vi "SubVI_TDMSfile_anal.vi"() -> (3 "file path out":path caption="파일 경로 출력")   [LabVIEW 2016]
uses:
  <vilib>/Utility/tdmsutil.llb/fileViewerConfigData.ctl
  <vilib>/Utility/error.llb/DialogType.ctl
  <vilib>/event_ctls.llb/sizeaction.ctl
  <vilib>/event_ctls.llb/panelstate.ctl
  <vilib>/Utility/tdmsutil.llb/TDMSFileViewerLocalizedText.vi
panel:
  out "Resize?":bool caption="크기 조정?"
  in  "Quit":bool caption="종료"
  in  "File contents":string(tree) caption="파일 내용"
  in  "Settings...":bool caption="셋팅..."
  in  "Status":string caption="상태"
  in  "Help":bool caption="도움말"
  in  "LastTopLeftValue":u64 caption="마지막 왼쪽 위 값"
  out "Temp Configuration":T1 caption="임시 설정"
  out "TotalCount":u64 caption="전체 카운트"
  out "error out":errorcluster caption="에러 출력"
  in  "error in (no error)":errorcluster caption="에러 입력(에러 없음)"
  in  "file path":path caption="파일 경로"
  in  "Properties / Values / Graph":T2(tab) caption="프로퍼티 / 값 / 그래프"
  in  "Properties":i32(listbox) caption="프로퍼티"
  in  "Go To":bool caption="이동하기"
  in  "Scrollbar":u64(c297) caption="스크롤 막대"
  in  "Raw data values":i32(listbox) caption="원시 데이터 값"
  out "dt":dbl
  out "Waveform Graph":waveform(dbl)[](graph) caption="웨이브폼 그래프"
  # "1...1000의 값을 디스플레이하기"
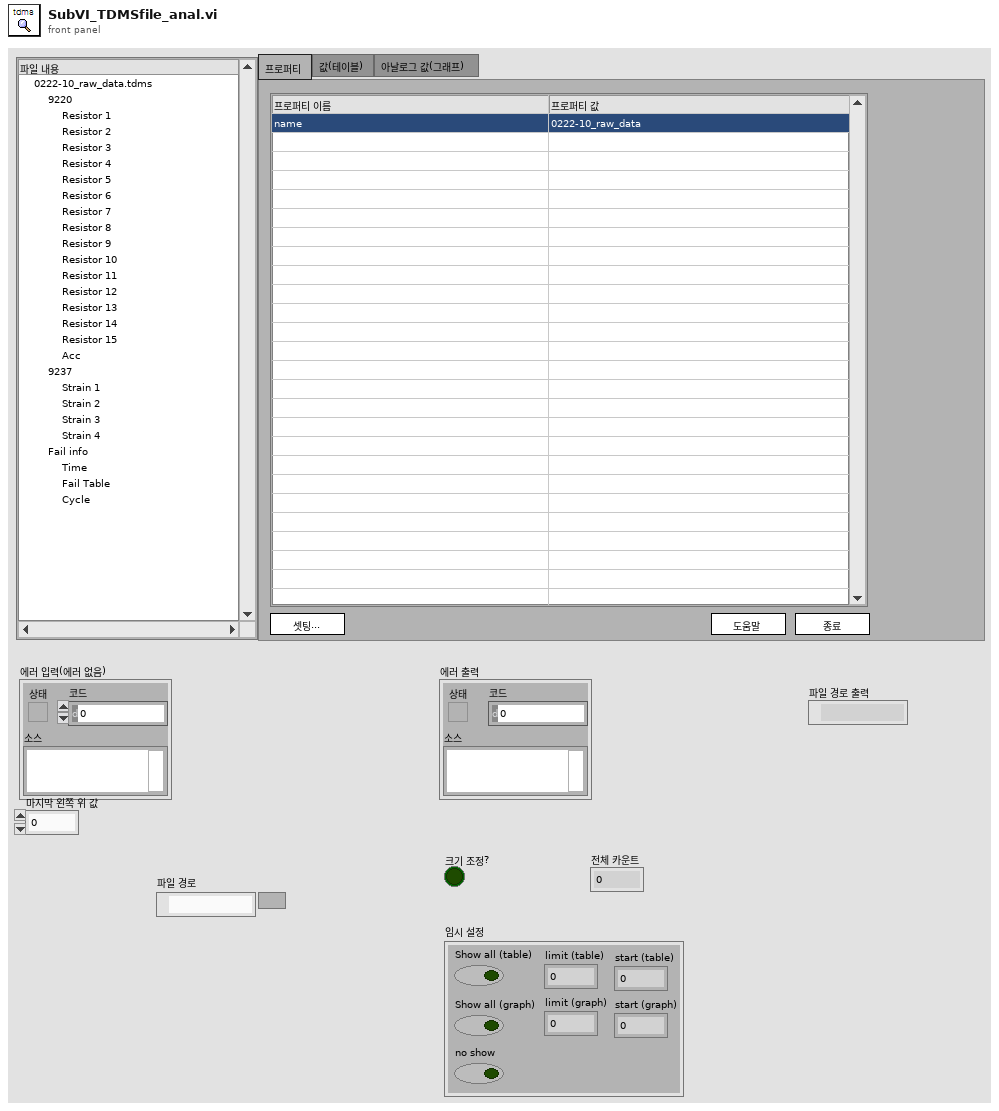
[diagram p1: front panel]
types:
  T1 = typedef "fileViewerConfigData.ctl" = cluster{"Show all (table)":bool, "Show all (graph)":bool, "limit (table)":u64, "limit (graph)":u64, "no show":bool, "start (table)":u64, "start (graph)":u64}
  T2 = enum32{"Properties", "Values (table)", "Analog values (graph)"}
  T3 = enum16{"open", "open or create", "create or replace", "create", "open (read-only)"}
  T4 = cluster{"Tree":refnum<vi>, "Tab Control":refnum<vi>, "property list":refnum<vi>, "raw data list":refnum<vi>, "Waveform Graph":refnum<vi>, "Ok":refnum<vi>, "Ok 2":refnum<vi>, "Ok 3":refnum<vi>, "Ok 4":refnum<vi>, "Scrollbar":refnum<vi>, "Ok 5":refnum<vi>, "TopLeftValue":refnum<vi>, "TotalCount":refnum<vi>}
  T5 = typedef "panelstate.ctl" = enum32{"Standard", "Minimized", "Maximized"}
  T6 = typedef "sizeaction.ctl" = enum32{"Minimized", "Maximized", "Resized"}
  T7 = cluster{"Shift":bool, "Ctrl":bool, "Alt":bool, "Cmd":bool, "Opt":bool}
  T8 = typedef "LVRectTypeDef.ctl" = cluster{"Left":i16, "Top":i16, "Right":i16, "Bottom":i16}
  T9 = typedef "LVRowAndColumnUnsignedTypeDef.ctl" = cluster{"Row":u32, "Column":u32}
  T10 = typedef "DialogType.ctl" = u16
  T11 = typedef "eventvkey.ctl" = enum16{"ASCII", "Enter", "Return", "Shift", "Ctrl", "Alt", "Cmd", "Opt", "Caps", "NumLock", "Clear", "Break", "Up", "Down", "Left", "Right", "Insert", "Delete", "Home", "End", "PageUp", "PageDown", "Escape", "Help", "Pause", "ScrollLock", "F1", "F2", "F3", "F4", "F5", "F6", "F7", "F8", "F9", "F10", "F11", "F12", "F13", "F14", "F15", "F16", "F17", "F18", "F19", "F20", "F21", "F22", "F23", "F24", "Play", "VolumeUp", "VolumeDown", "Mute", "Two Byte Char"}
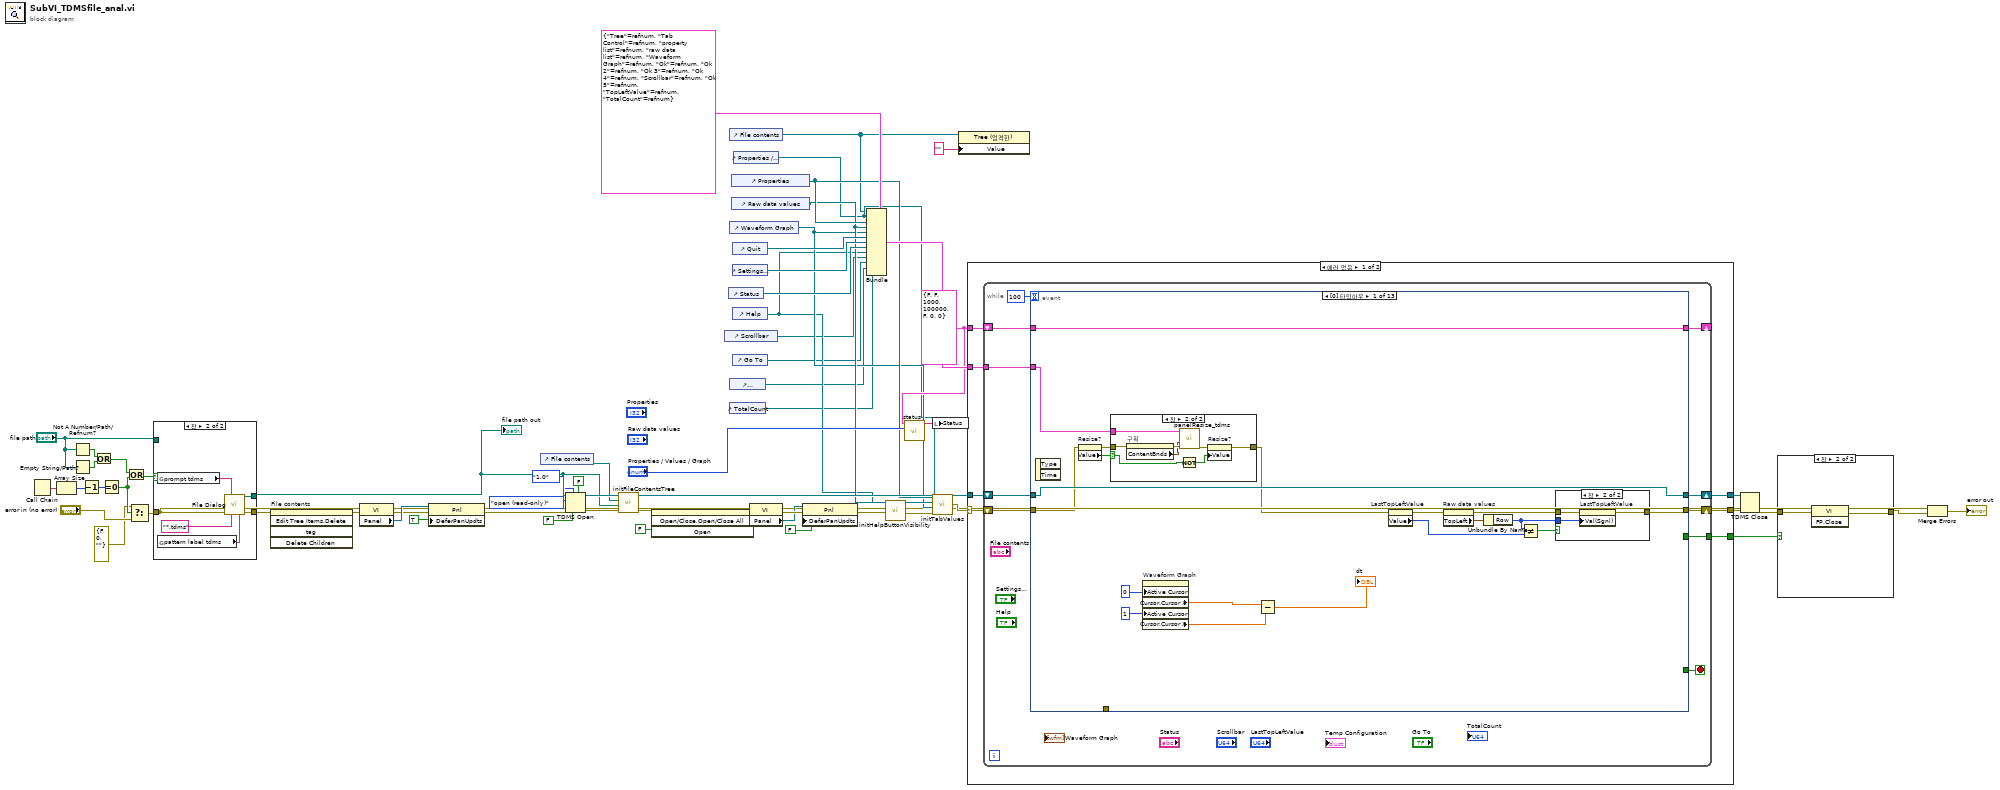
[diagram p0: block diagram]
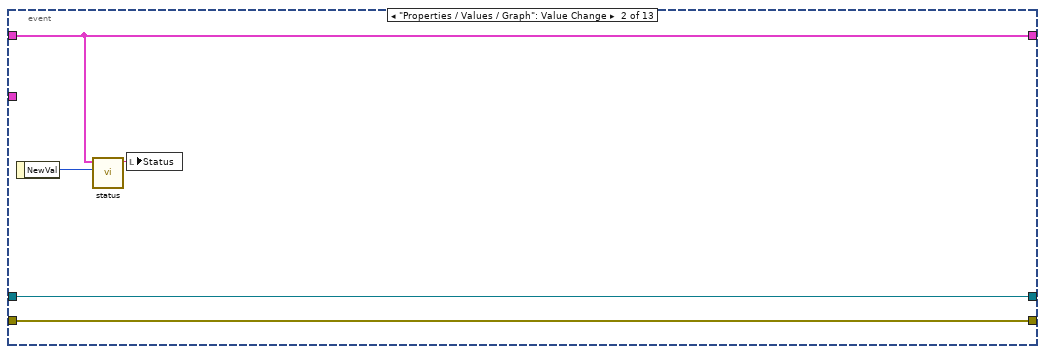
[diagram p5: hidden frame]
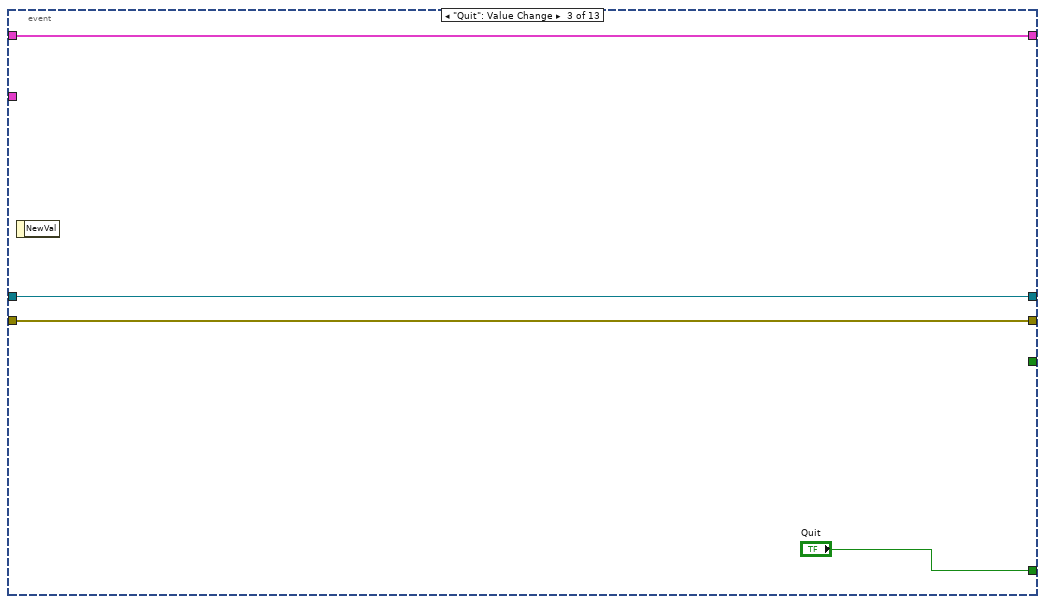
[diagram p6: hidden frame]
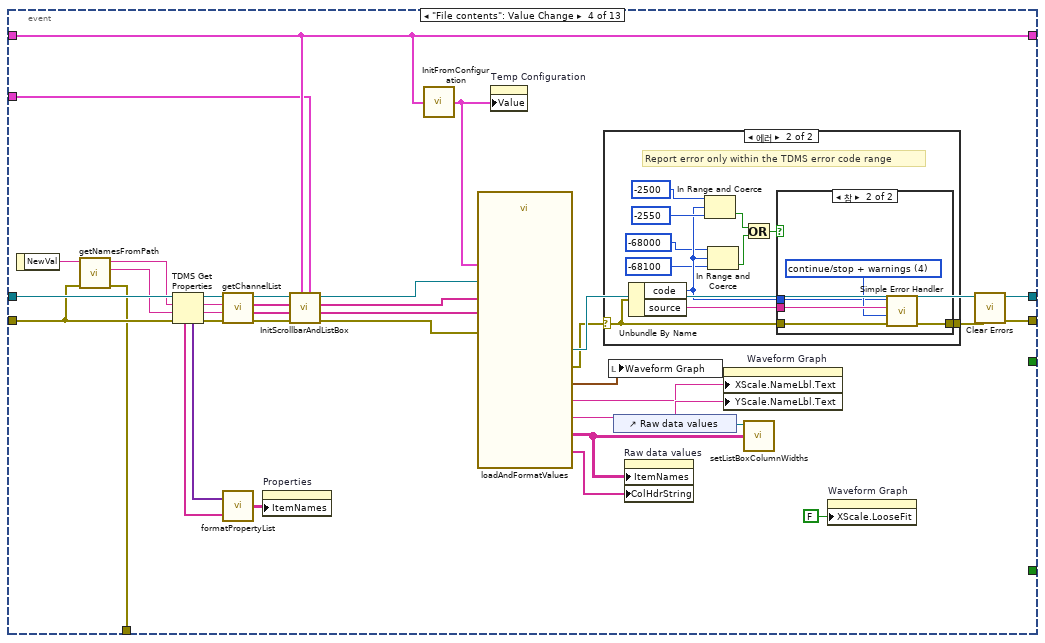
[diagram p7: hidden frame]
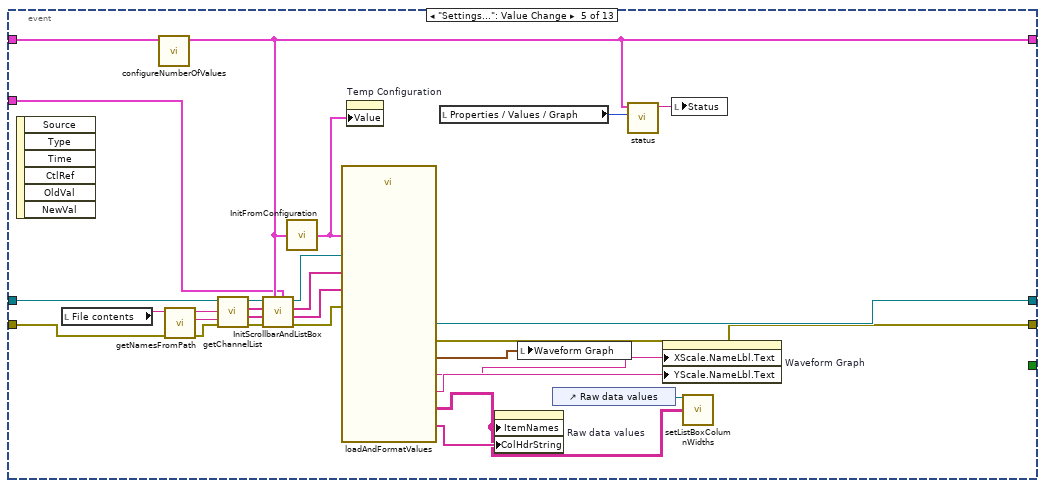
[diagram p10: hidden frame]
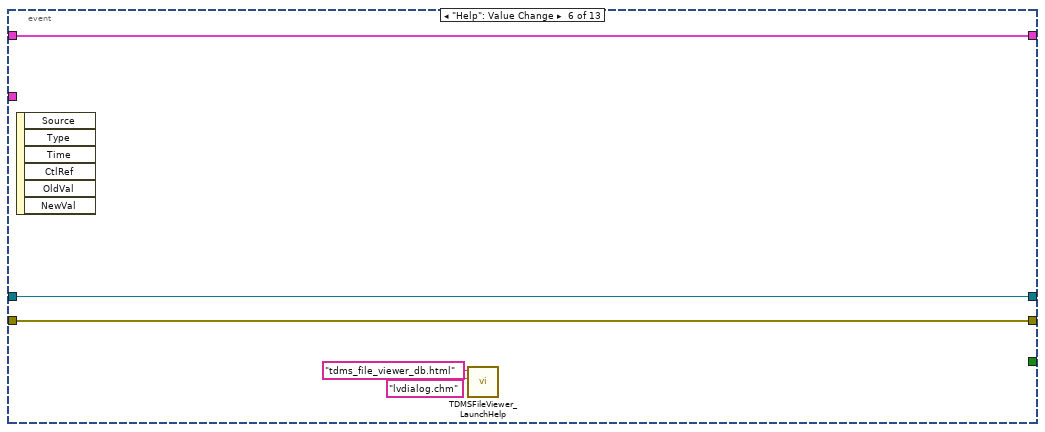
[diagram p11: hidden frame]
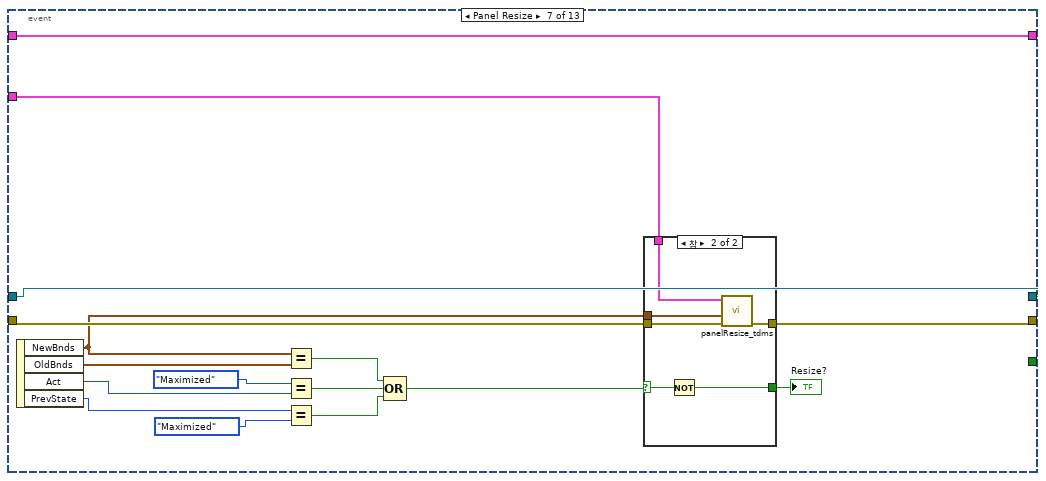
[diagram p12: hidden frame]
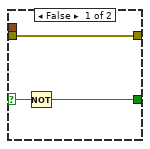
[diagram p13: hidden frame]
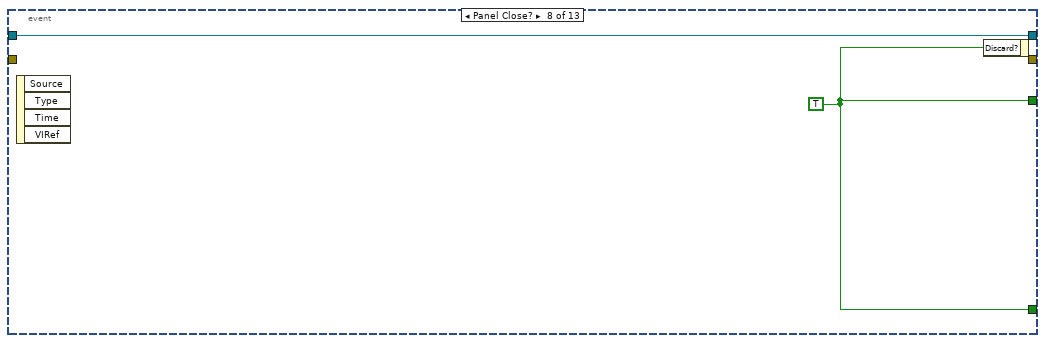
[diagram p14: hidden frame]
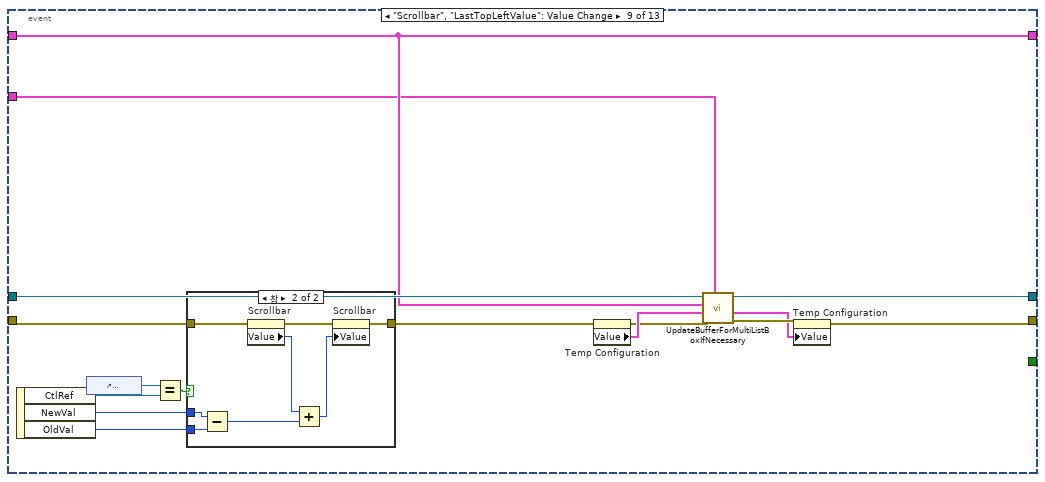
[diagram p15: hidden frame]
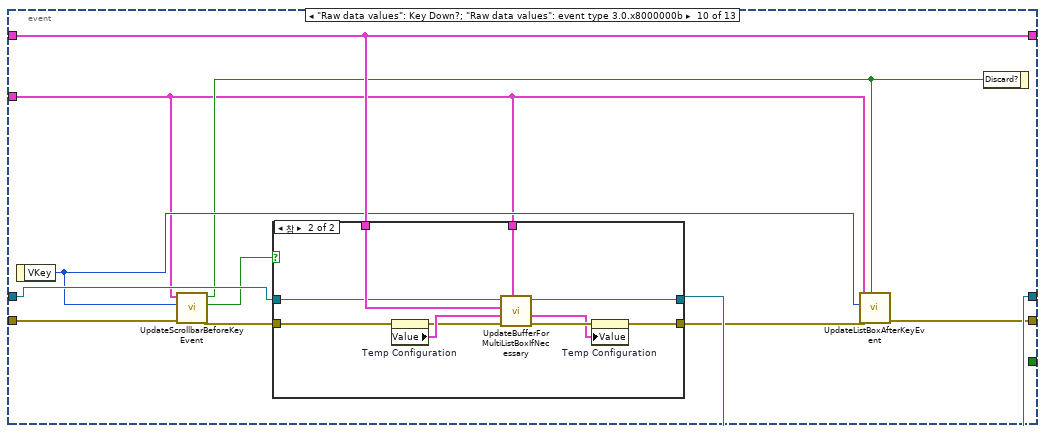
[diagram p17: hidden frame]
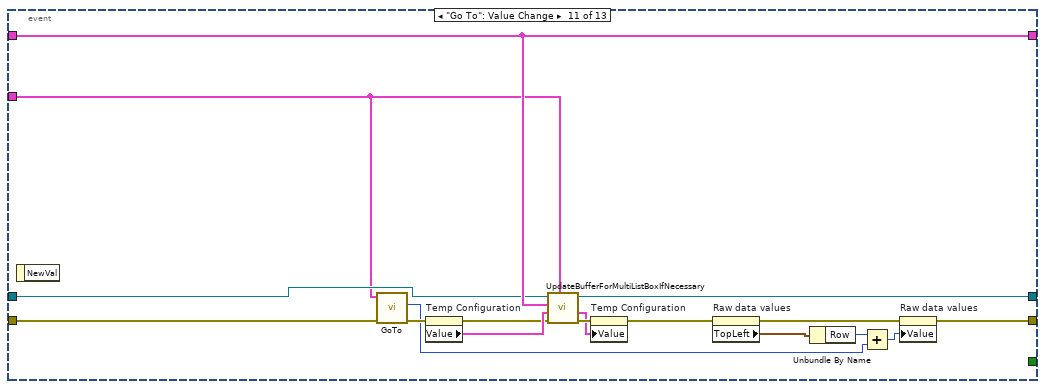
[diagram p19: hidden frame]
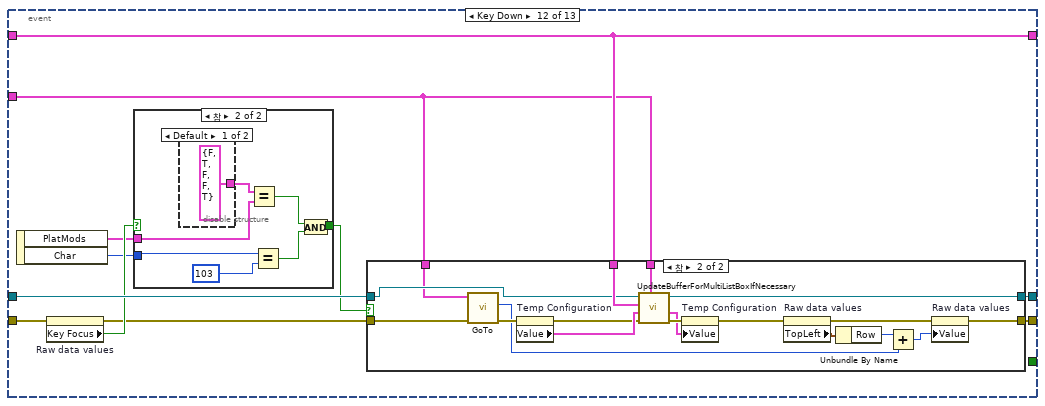
[diagram p20: hidden frame]
diagram:
  w27 = T1 {"Show all (table)"=FALSE, "Show all (graph)"=FALSE, "limit (table)"=1000, "limit (graph)"=100000, "no show"=FALSE, "start (table)"=0, "start (graph)"=0} ("TDMS File Viewer Configuration")
  n1 = Call Chain() -> (call chain=w42:string[])
  n2 = Array Size(array=w42) -> (size(s)=w40:i32)
  n3 = Not A Number/Path/Refnum?(number/path/refnum="file path") -> (NaN/Path/Refnum?=w44:bool)
  n4 = Empty String/Path?(string/path="file path") -> (empty?=w43:bool)
  n5 = Decrement(x=w40) -> (x-1=w39:i32)
  n6 = Or(x=w44, y=w43) -> (x .or. y?=w41:bool)
  n7 = Equal To 0?(x=w39) -> (x = 0?=w25:bool)
  n8 = Or(x=w41, y=w25) -> (x .or. y?=w38:bool)
  n9 = Select(t=errorcluster {"status"=FALSE, "code"=0, "source"=""}, s=w25, f="error in (no error)") -> (s? t:f=w6:errorcluster)
  n10 = case shown="참" w38 {
    tunnel: [w63 w69] -> w31
    tunnel: "file path" -> [w63 _]
    tunnel: [w62 w67] -> w30
    tunnel: w6 -> [w62 w66]
    frame False {
    }
    frame True {
      n11 = global read "TDMSFileViewerLocalizedText.vi" "prompt tdms"() -> (w65:string)
      n12 = global read "TDMSFileViewerLocalizedText.vi" "pattern label tdms"() -> (w64:string)
      n13 = call "File Dialog"("prompt"=w65, "error in"=w66, "pattern (all files)"="*.tdms", "pattern label"=w64) -> ("selected path"=w69:path, "error out"=w67:errorcluster)  [unwired: 3 in, 7 out]
    }
  }
  "file path out" <- w31
  n14 = invoke on="File contents" class="Tree (strict)" method="Edit Tree Items.Delete"(error in=w30) -> (error out=w52:errorcluster)  [unwired: 4 in, 4 out]
  n15 = property class="VI"(error in=w52) -> (error out=w53:errorcluster, "Panel"=w54:refnum<vi>)  [unwired: 1 in, 1 out]
  n16 = property class="Pnl"(reference=w54, error in=w53, "DeferPanUpdts"=TRUE ("Defer Panel Updates")) -> (error out=w56:errorcluster)  [unwired: 1 out]
  n17 = control-ref of="File contents"() -> (w32:refnum<vi>)
  n18 = TDMS Open(5:FALSE ("create index file? (T)"), 6:FALSE ("disable buffering (T)"), 7:enum16{"1.0", "2.0"}."1.0" ("file format version (2.0)"), 8:w56, 10:T3."open (read-only)" ("operation"), 11:w31) -> (0:w61:errorcluster, 3:w60:refnum<k34>)  [unwired: 1 in]
  n19 = call <vilib>:"initFileContentsTree.vi"("error in (no error)"=w61, "file path"=w31, "Tree Refnum"=w32, "tdms file"=w60) -> ("error out"=w48:errorcluster, "tdms file out"=w59:refnum<k34>)  [unwired: 2 out]
  n20 = invoke on="File contents" class="Tree (strict)" method="Open/Close.Open/Close All"(error in=w48, "Open"=FALSE ("Open?")) -> (error out=w47:errorcluster)  [unwired: 2 in, 3 out]
  n21 = control-ref of="Scrollbar"() -> (w5:refnum<vi>)
  n22 = control-ref of="Status"() -> (w29:refnum<vi>)
  n23 = control-ref of="File contents"() -> (w13:refnum<vi>)
  n24 = control-ref of="Waveform Graph"() -> (w15:refnum<vi>)
  n25 = control-ref of="LastTopLeftValue"() -> (w3:refnum<vi>)
  n26 = control-ref of="TotalCount"() -> (w2:refnum<vi>)
  n27 = control-ref of="Properties"() -> (w17:refnum<vi>)
  n28 = control-ref of="Raw data values"() -> (w16:refnum<vi>)
  n29 = control-ref of="Quit"() -> (w36:refnum<vi>)
  n30 = control-ref of="Settings..."() -> (w34:refnum<vi>)
  n31 = control-ref of="Help"() -> (w9:refnum<vi>)
  n32 = control-ref of="Go To"() -> (w4:refnum<vi>)
  n33 = control-ref of="Properties / Values / Graph"() -> (w14:refnum<vi>)
  n34 = property class="VI"(error in=w47) -> (error out=w50:errorcluster, "Panel"=w49:refnum<vi>)  [unwired: 1 in, 1 out]
  n35 = property class="Pnl"(reference=w49, error in=w50, "DeferPanUpdts"=FALSE ("Defer Panel Updates")) -> (error out=w11:errorcluster)  [unwired: 1 out]
  n36 = Bundle(cluster=T4 {"Tree"=refnum, "Tab Control"=refnum, "property list"=refnum, "raw data list"=refnum, "Waveform Graph"=refnum, "Ok"=refnum, "Ok 2"=refnum, "Ok 3"=refnum, "Ok 4"=refnum, "Scrollbar"=refnum, "Ok 5"=refnum, "TopLeftValue"=refnum, "TotalCount"=refnum} ("control refs"), "Tree"=w13, "Tab Control"=w14, "property list"=w17, "raw data list"=w16, "Waveform Graph"=w15, "Ok"=w36, "Ok 2"=w34, "Ok 3"=w29, "Ok 4"=w9, "Scrollbar"=w5, "Ok 5"=w4, "TopLeftValue"=w3, "TotalCount"=w2) -> (w37:T4)
  n37 = call <vilib>:"initHelpButtonVisibility.vi"("error in"=w11, "Help"=w9) -> ("error out"=w10:errorcluster)  [unwired: 9 in]
  n38 = call <vilib>:"status.vi"("tab sheet"="Properties / Values / Graph", "TDMS File Viewer Configuration"=w27) -> ("status"=w28:string)  [unwired: 5 out]
  n39 = local write "Status"(w28) -> ()
  n40 = call <vilib>:"initTabValues.vi"("properties"=w17, "Values"=w16, "waveform"=w15, "error in"=w10, "Properties / Values / Graph"=w14) -> ("error out"=w18:errorcluster)
  n41 = property class="Tree (엄격한)"(reference=w13, "Value"="") -> ()  [unwired: 1 in, 2 out]
  n42 = case shown="에러 없음" w18 {
    selector: w18 -> [w71 w358]
    tunnel: w59 -> [w76 w359]
    tunnel: [w75 w359] -> w58
    tunnel: [w74 w357] -> w57
    tunnel: w37 -> [w73 _]
    tunnel: w27 -> [w72 _]
    tunnel: [w70 FALSE] -> w22
    frame No Error {
      n43 = while {
        shift-right: [w84] -> w74
        shift-left: w71 -> [w85]
        shift-right: [w83] -> w75
        shift-left: w76 -> [w86]
        tunnel: w73 -> [w81]
        shift-right: [w79] -> _
        shift-left: w72 -> [w80]
        tunnel: [w78] -> w70
        stop <- w82 stop-if-true
        n44 = event shown="[0] 타임아웃" {
          selector: _ -> [_ _ _ _ _ _ _ _ _ _ _ _ _]
          dyn-events: _ -> [_ _ _ _ _ _ _ _ _ _ _ _ _]
          timeout: 100 -> [_ _ _ _ _ _ _ _ _ _ _ _ _]
          tunnel: w86 -> [w105 w122 w126 w162 w197 w212 w229 w240 w256 w275 w300 w315 w348]
          tunnel: w85 -> [w100 w123 w125 w154 w205 w211 w227 _ w243 w267 w289 w312 w347]
          tunnel: [w93 w123 w125 w150 w206 w211 w226 _ w250 w272 w292 w313 w347] -> w84
          tunnel: [w105 w122 w126 w161 w207 w212 w229 w240 w255 w274 w299 w314 w348] -> w83
          tunnel: [_ _ "Quit" _ _ _ _ w239 _ _ _ _ _] -> w82
          tunnel: [_ _ _ w153 _ _ _ _ _ _ _ _ _] -> _
          tunnel: w81 -> [w101 _ _ w128 w181 _ w228 _ w242 w268 w290 w309 _]
          tunnel: w80 -> [w104 w119 w124 w129 w208 w213 w225 _ w254 w276 w301 w316 w349]
          tunnel: [w104 w119 w124 w129 w183 w213 w225 _ w254 w276 w301 w316 w349] -> w79
          tunnel: [_ _ _ _ _ _ _ w239 _ _ _ _ _] -> w78
          event Timeout {
            n45 = event-data() -> ()  [unwired: 3 out]
            n46 = property on="Resize?" class="Bool (엄격한)"(error in=w100) -> (error out=w102:errorcluster, "Value"=w103:bool)  [unwired: 1 in, 1 out]
            n47 = case shown="참" w103 {
              selector: w103 -> [_ w117]
              tunnel: w101 -> [_ w118]
              tunnel: w102 -> [w110 w113]
              tunnel: [w110 w115] -> w98
              frame False {
              }
              frame True {
                n48 = property on="구획" class="Pane"(error in=w113) -> (error out=w112:errorcluster, "ContentBnds"=w111:T8)  [unwired: 1 in, 1 out]
                n49 = Not(x=w117) -> (.not. x?=w114:bool)
                n50 = call <vilib>:"panelResize_tdms.vi"("error in (no error)"=w112, "NewBnds"=w111, "control refs"=w118) -> ("error out"=w116:errorcluster)  [unwired: 4 in]
                n51 = property on="Resize?" class="Bool (엄격한)"(error in=w116, "Value"=w114) -> (error out=w115:errorcluster)  [unwired: 1 in, 1 out]
              }
            }
            n52 = property on="Waveform Graph" class="WFGraph (엄격한)"("Active Cursor"=u32 0 ("활성 커서"), "Active Cursor"=u32 1 ("활성 커서")) -> ("Cursor.Cursor X"=w89:dbl, "Cursor.Cursor X"=w88:dbl)  [unwired: 2 in, 2 out]
            n53 = Subtract(x=w89, y=w88) -> (x-y=→"dt":dbl)
            n54 = property on="LastTopLeftValue" class="DigNum (엄격한)"(error in=w98) -> (error out=w97:errorcluster, "Value"=w96:u64)  [unwired: 1 in, 1 out]
            n55 = property on="Raw data values" class="MCListbox (엄격한)"(error in=w97) -> (error out=w94:errorcluster, "TopLeft"=w99:T9)  [unwired: 1 in, 1 out]
            n56 = Unbundle By Name(w99) -> ("Row"=w92:u32)
            n57 = Not Equal?(x=w92, y=w96) -> (x != y?=w95:bool)
            n58 = case shown="참" w95 {
              tunnel: w94 -> [w106 w109]
              tunnel: [w106 w108] -> w93
              tunnel: w92 -> [_ w107]
              frame False {
              }
              frame True {
                n59 = property on="LastTopLeftValue" class="DigNum (엄격한)"(error in=w109, "Val(Sgnl)"=w107) -> (error out=w108:errorcluster)  [unwired: 1 in, 1 out]
              }
            }
          }
          event "Properties / Values / Graph": Value Change {
            n60 = event-data() -> ("NewVal"=w121:T2)  [unwired: 1 out]
            n61 = call <vilib>:"status.vi"("tab sheet"=w121, "TDMS File Viewer Configuration"=w119) -> ("status"=w120:string)  [unwired: 5 out]
            n62 = local write "Status"(w120) -> ()
          }
          event "Quit": Value Change {
            n63 = event-data() -> ()  [unwired: 2 out]
          }
          event "File contents": Value Change {
            n64 = event-data() -> ("NewVal"=w156:string)  [unwired: 1 out]
            n65 = call <vilib>:"getNamesFromPath.vi"("error in (no error)"=w154, "tree path"=w156) -> ("error out"=w153:errorcluster, "channel"=w159:string, "group"=w160:string)  [unwired: 3 out]
            n66 = TDMS Get Properties(8:w154, 9:w159, 10:w160, 11:w162) -> (0:w148:errorcluster, 1:w147:string, 2:w142:string, 3:w149:refnum<k34>, 4:w157:variant[], 6:w158:string[])  [unwired: 2 out]
            n67 = call <vilib>:"getChannelList.vi"("error in (no error)"=w148, "channel names"=w147, "group name"=w142, "tdms file"=w149) -> ("error out"=w137:errorcluster, "channel names out"=w135:string[], "group names out"=w133:string[], "tdms file out"=w131:refnum<k34>)
            n68 = call <vilib>:"formatPropertyList.vi"("property names"=w158, "property values"=w157) -> ("strings"=w155:string[][])
            n69 = property on="Properties" class="MCListbox (엄격한)"("ItemNames"=w155) -> ()  [unwired: 2 in, 2 out]
            n70 = call <vilib>:"InitScrollbarAndListBox.vi"("control refs"=w128, "configuration"=w129, "error in (no error)"=w137, "channel names"=w135, "group names"=w133, "tdms in"=w131) -> ("error out"=w136:errorcluster, "channel out"=w134:string[], "group out"=w132:string[], "tdms out"=w130:refnum<k34>)  [unwired: 2 in]
            n71 = call <vilib>:"InitFromConfiguration.vi"("configuration"=w129) -> ("output cluster"=w138:T1)  [unwired: 4 in]
            n72 = call <vilib>:"loadAndFormatValues.vi"("error in (no error)"=w136, "configuration"=w138, "channel names"=w134, "group names"=w132, "tdms file"=w130) -> ("error out"=w141:errorcluster, "graph y names"=w145:string, "graph x names"=w144:string, "tdms file out"=w161:refnum<k34>, "waveform values"=w143:waveform(dbl)[], "table values"=w152:string[][], "table headers"=w146:string[])
            n73 = property on="Temp Configuration" class="Clust (엄격한)"("Value"=w138) -> ()  [unwired: 2 in, 2 out]
            n74 = case shown="에러" w141 {
              selector: w141 -> [w163 w173]
              tunnel: [w163 w172] -> w140
              frame No Error {
              }
              frame Error {
                # "Report error only within the TDMS error code range"
                n75 = Unbundle By Name(w173) -> ("code"=w169:i32, "source"=w174:string)
                n76 = In Range and Coerce(upper limit=-2500, x=w169, lower limit=-2550 ("upper limit")) -> (In Range?=w166:bool)  [unwired: 1 out]
                n77 = In Range and Coerce(upper limit=-68000, x=w169, lower limit=-68100) -> (In Range?=w165:bool)  [unwired: 1 out]
                n78 = Or(x=w166, y=w165) -> (x .or. y?=w164:bool)
                n79 = case shown="참" w164 {
                  tunnel: w174 -> [_ w180]
                  tunnel: w173 -> [w175 w179]
                  tunnel: [w175 w178] -> w172
                  tunnel: w169 -> [_ w176]
                  frame False {
                    # "Out of the range of TDMS\nerror code, we don't report\nthem."
                  }
                  frame True {
                    w177 = T10 4 items=["no dialog", "OK message", "continue or stop message", "OK message + warnings", "continue/stop + warnings"] ("type of dialog (OK msg:1)")
                    n80 = call <vilib>:"Simple Error Handler.vi"("error code (no error:0)"=w176, "error source (\" \")"=w180, "type of dialog (OK msg:1)"=w177, "error in (no error)"=w179) -> ("error out"=w178:errorcluster)  [unwired: 1 in, 4 out]
                  }
                }
              }
            }
            n81 = local write "Waveform Graph"(w143) -> ()
            n82 = control-ref of="Raw data values"() -> (w151:refnum<vi>)
            n83 = property on="Raw data values" class="MCListbox (엄격한)"("ItemNames"=w152, "ColHdrString"=w146) -> ()  [unwired: 2 in, 2 out]
            n84 = property on="Waveform Graph" class="WFGraph (엄격한)"("XScale.NameLbl.Text"=w144, "YScale.NameLbl.Text"=w145) -> ()  [unwired: 2 in, 2 out]
            n85 = call <vilib>:"setListBoxColumnWidths.vi"("table data"=w152, "MCListbox Refnum"=w151) -> ()  [unwired: 1 out]
            n86 = property on="Waveform Graph" class="WFGraph (엄격한)"("XScale.LooseFit"=FALSE ("X Scale.Loose Fit")) -> ()  [unwired: 2 in, 2 out]
            n87 = call <vilib>:"Clear Errors.vi"("error in (no error)"=w140) -> ("error out"=w150:errorcluster)  [unwired: 1 in, 5 out]
          }
          event "Settings...": Value Change {
            n88 = event-data() -> ()  [unwired: 7 out]
            n89 = local read "File contents"() -> (w198:string)
            n90 = call <vilib>:"configureNumberOfValues.vi"("TDMS File Viewer Configuration"=w208) -> ("TDMS File Viewer Configuration Out"=w183:T1)  [unwired: 10 out]
            n91 = call <vilib>:"getNamesFromPath.vi"("error in (no error)"=w205, "tree path"=w198) -> ("error out"=w196:errorcluster, "channel"=w194:string, "group"=w195:string)  [unwired: 3 out]
            n92 = call <vilib>:"getChannelList.vi"("error in (no error)"=w196, "channel names"=w194, "group name"=w195, "tdms file"=w197) -> ("error out"=w185:errorcluster, "channel names out"=w187:string[], "group names out"=w189:string[], "tdms file out"=w191:refnum<k34>)
            n93 = call <vilib>:"InitScrollbarAndListBox.vi"("control refs"=w181, "configuration"=w183, "error in (no error)"=w185, "channel names"=w187, "group names"=w189, "tdms in"=w191) -> ("error out"=w184:errorcluster, "channel out"=w186:string[], "group out"=w188:string[], "tdms out"=w190:refnum<k34>)  [unwired: 2 in]
            n94 = call <vilib>:"InitFromConfiguration.vi"("configuration"=w183) -> ("output cluster"=w182:T1)  [unwired: 4 in]
            n95 = call <vilib>:"loadAndFormatValues.vi"("error in (no error)"=w184, "configuration"=w182, "channel names"=w186, "group names"=w188, "tdms file"=w190) -> ("error out"=w206:errorcluster, "graph y names"=w200:string, "graph x names"=w199:string, "tdms file out"=w207:refnum<k34>, "waveform values"=w204:waveform(dbl)[], "table values"=w201:string[][], "table headers"=w203:string[])
            n96 = property on="Temp Configuration" class="Clust (엄격한)"("Value"=w182) -> ()  [unwired: 2 in, 2 out]
            n97 = local read "Properties / Values / Graph"() -> (w192:T2)
            n98 = property on="Raw data values" class="MCListbox (엄격한)"("ItemNames"=w201, "ColHdrString"=w203) -> ()  [unwired: 2 in, 2 out]
            n99 = local write "Waveform Graph"(w204) -> ()
            n100 = control-ref of="Raw data values"() -> (w202:refnum<vi>)
            n101 = call <vilib>:"status.vi"("tab sheet"=w192, "TDMS File Viewer Configuration"=w183) -> ("status"=w193:string)  [unwired: 5 out]
            n102 = property on="Waveform Graph" class="WFGraph (엄격한)"("XScale.NameLbl.Text"=w199, "YScale.NameLbl.Text"=w200) -> ()  [unwired: 2 in, 2 out]
            n103 = local write "Status"(w193) -> ()
            n104 = call <vilib>:"setListBoxColumnWidths.vi"("table data"=w201, "MCListbox Refnum"=w202) -> ()  [unwired: 1 out]
          }
          event "Help": Value Change {
            n105 = event-data() -> ()  [unwired: 7 out]
            n106 = call <vilib>:"TDMSFileViewer_LaunchHelp.vi"("CHM or HLP filename (lvdialog.chm)"="lvdialog.chm", "HTML filename"="tdms_file_viewer_db.html") -> ()  [unwired: 1 in, 5 out]
          }
          event Panel Resize {
            n107 = event-data() -> ("NewBnds"=w217:T8, "OldBnds"=w216:T8, "Act"=w218:T6, "PrevState"=w219:T5)  [unwired: 1 out]
            n108 = Equal?(x=w217, y=w216) -> (x = y?=w222:bool)
            n109 = Equal?(x=sizeaction."Maximized" ("Act"), y=w218) -> (x = y?=w221:bool)
            n110 = Equal?(x=w219, y=panelstate."Maximized" ("PrevState")) -> (x = y?=w220:bool)
            n111 = Compound Arithmetic op=OR(w222, w221, w220) -> (w215:bool)
            n112 = case shown="참" w215 {
              selector: w215 -> [w231 w234]
              tunnel: w228 -> [_ w238]
              tunnel: w227 -> [w232 w237]
              tunnel: [w232 w236] -> w226
              tunnel: w217 -> [_ w235]
              tunnel: [w230 w233] -> w214
              frame False {
                n113 = Not(x=w231) -> (.not. x?=w230:bool)
              }
              frame True {
                n114 = Not(x=w234) -> (.not. x?=w233:bool)
                n115 = call <vilib>:"panelResize_tdms.vi"("error in (no error)"=w237, "NewBnds"=w235, "control refs"=w238) -> ("error out"=w236:errorcluster)  [unwired: 4 in]
              }
            }
            "Resize?" <- w214
          }
          event Panel Close? {
            w239 = TRUE
            n116 = event-data() -> ()  [unwired: 5 out]
            n117 = event-data("Discard?"=w239) -> ()  [unwired: 1 in, 1 out]
          }
          event "Scrollbar", "LastTopLeftValue": Value Change {
            n118 = event-data() -> ("CtlRef"=w248:refnum<vi>, "NewVal"=w245:u64, "OldVal"=w244:u64)  [unwired: 1 out]
            n119 = control-ref of="LastTopLeftValue"() -> (w247:refnum<vi>)
            n120 = Equal?(x=w247, y=w248) -> (x = y?=w246:bool)
            n121 = case shown="참" w246 {
              tunnel: w245 -> [_ w261]
              tunnel: w244 -> [_ w260]
              tunnel: w243 -> [w257 w259]
              tunnel: [w257 w258] -> w241
              frame False {
              }
              frame True {
                n122 = Subtract(x=w261, y=w260) -> (x-y=w263:u64)
                n123 = property on="Scrollbar" class="Scroll (엄격한)"(error in=w259) -> (error out=w265:errorcluster, "Value"=w264:u64)  [unwired: 1 in, 1 out]
                n124 = Add(x=w264, y=w263) -> (x+y=w262:u64)
                n125 = property on="Scrollbar" class="Scroll (엄격한)"(error in=w265, "Value"=w262) -> (error out=w258:errorcluster)  [unwired: 1 in, 1 out]
              }
            }
            n126 = property on="Temp Configuration" class="Clust (엄격한)"(error in=w241) -> (error out=w252:errorcluster, "Value"=w253:T1)  [unwired: 1 in, 1 out]
            n127 = call <vilib>:"UpdateBufferForMultiListBoxIfNecessary.vi"("control refs"=w242, "error in"=w252, "Buffer Configuration"=w253, "TDMS File Viewer Configuration"=w254, "tdms file in"=w256) -> ("error out"=w251:errorcluster, "BufferConfig out"=w249:T1, "tdms file out"=w255:refnum<k34>)  [unwired: 4 in]
            n128 = property on="Temp Configuration" class="Clust (엄격한)"(error in=w251, "Value"=w249) -> (error out=w250:errorcluster)  [unwired: 1 in, 1 out]
          }
          event "Raw data values": Key Down?; "Raw data values": event type 3.0.x8000000b {
            n129 = event-data() -> ("VKey"=w270:T11)  [unwired: 1 out]
            n130 = call <vilib>:"UpdateScrollbarBeforeKeyEvent.vi"("error in (no error)"=w267, "VKey"=w270, "control refs 2"=w268) -> ("error out"=w273:errorcluster, "LoadBuffer?"=w271:bool, "DiscardEvent?"=w269:bool)  [unwired: 6 in]
            n131 = case shown="참" w271 {
              tunnel: w276 -> [_ w284]
              tunnel: w275 -> [w277 w283]
              tunnel: [w277 w282] -> w274
              tunnel: w273 -> [w278 w279]
              tunnel: [w278 w281] -> w266
              tunnel: w268 -> [_ w280]
              frame False {
              }
              frame True {
                n132 = property on="Temp Configuration" class="Clust (엄격한)"(error in=w279) -> (error out=w287:errorcluster, "Value"=w288:T1)  [unwired: 1 in, 1 out]
                n133 = call <vilib>:"UpdateBufferForMultiListBoxIfNecessary.vi"("control refs"=w280, "error in"=w287, "Buffer Configuration"=w288, "TDMS File Viewer Configuration"=w284, "tdms file in"=w283) -> ("error out"=w286:errorcluster, "BufferConfig out"=w285:T1, "tdms file out"=w282:refnum<k34>)  [unwired: 4 in]
                n134 = property on="Temp Configuration" class="Clust (엄격한)"(error in=w286, "Value"=w285) -> (error out=w281:errorcluster)  [unwired: 1 in, 1 out]
              }
            }
            n135 = call <vilib>:"UpdateListBoxAfterKeyEvent.vi"("DiscardEvent?"=w269, "error in (no error)"=w266, "VKey"=w270, "control refs"=w268) -> ("error out"=w272:errorcluster)  [unwired: 7 in]
            n136 = event-data("Discard?"=w269) -> ()  [unwired: 1 in, 1 out]
          }
          event "Go To": Value Change {
            n137 = event-data() -> ()  [unwired: 2 out]
            n138 = call <vilib>:"GoTo.vi"("error in"=w289, "control refs"=w290) -> ("error out"=w298:errorcluster, "VisibleValue"=w295:u64)  [unwired: 8 in]
            n139 = property on="Temp Configuration" class="Clust (엄격한)"(error in=w298) -> (error out=w304:errorcluster, "Value"=w305:T1)  [unwired: 1 in, 1 out]
            n140 = call <vilib>:"UpdateBufferForMultiListBoxIfNecessary.vi"("control refs"=w290, "error in"=w304, "Buffer Configuration"=w305, "TDMS File Viewer Configuration"=w301, "tdms file in"=w300) -> ("error out"=w303:errorcluster, "BufferConfig out"=w302:T1, "tdms file out"=w299:refnum<k34>)  [unwired: 4 in]
            n141 = property on="Temp Configuration" class="Clust (엄격한)"(error in=w303, "Value"=w302) -> (error out=w291:errorcluster)  [unwired: 1 in, 1 out]
            n142 = property on="Raw data values" class="MCListbox (엄격한)"(error in=w291) -> (error out=w293:errorcluster, "TopLeft"=w297:T9)  [unwired: 1 in, 1 out]
            n143 = Unbundle By Name(w297) -> ("Row"=w296:u32)
            n144 = Add(x=w296, y=w295) -> (x+y=w294:u64)
            n145 = property on="Raw data values" class="MCListbox (엄격한)"(error in=w293, "Value"=w294) -> (error out=w292:errorcluster)  [unwired: 1 in, 1 out]
          }
          event Key Down {
            n146 = event-data() -> ("PlatMods"=w308:T7, "Char"=w307:i16)  [unwired: 1 out]
            n147 = property on="Raw data values" class="MCListbox (엄격한)"(error in=w312) -> (error out=w306:errorcluster, "Key Focus"=w311:bool)  [unwired: 1 in, 1 out]
            n148 = case shown="참" w311 {
              selector: w311 -> [w317 _]
              tunnel: [w317 w318] -> w310
              tunnel: w308 -> [_ w323]
              tunnel: w307 -> [_ w322]
              frame False {
              }
              frame True {
                n149 = disable-structure shown="Default" {
                  disable-tunnel: [T7 {"Shift"=FALSE, "Ctrl"=TRUE, "Alt"=FALSE, "Cmd"=FALSE, "Opt"=TRUE} ("PlatMods") T7 {"Shift"=FALSE, "Ctrl"=FALSE, "Alt"=FALSE, "Cmd"=TRUE, "Opt"=FALSE} ("PlatMods")] -> w324
                  frame condition #0 (active) {
                  }
                  frame condition #1 {
                  }
                }
                n150 = Equal?(x=w324, y=w323) -> (x = y?=w320:bool)
                n151 = Equal?(x=w322, y=i16 103 ("Char")) -> (x = y?=w319:bool)
                n152 = And(x=w320, y=w319) -> (x .and. y?=w318:bool)
              }
            }
            n153 = case shown="참" w310 {
              tunnel: w316 -> [_ w342]
              tunnel: w315 -> [w327 w341]
              tunnel: [w327 w340] -> w314
              tunnel: [w328 w333] -> w313
              tunnel: w306 -> [w328 w329]
              tunnel: w309 -> [_ w331]
              tunnel: w309 -> [_ w330]
              frame False {
              }
              frame True {
                n154 = call <vilib>:"GoTo.vi"("error in"=w329, "control refs"=w330) -> ("error out"=w339:errorcluster, "VisibleValue"=w336:u64)  [unwired: 8 in]
                n155 = property on="Temp Configuration" class="Clust (엄격한)"(error in=w339) -> (error out=w345:errorcluster, "Value"=w346:T1)  [unwired: 1 in, 1 out]
                n156 = call <vilib>:"UpdateBufferForMultiListBoxIfNecessary.vi"("control refs"=w331, "error in"=w345, "Buffer Configuration"=w346, "TDMS File Viewer Configuration"=w342, "tdms file in"=w341) -> ("error out"=w344:errorcluster, "BufferConfig out"=w343:T1, "tdms file out"=w340:refnum<k34>)  [unwired: 4 in]
                n157 = property on="Temp Configuration" class="Clust (엄격한)"(error in=w344, "Value"=w343) -> (error out=w332:errorcluster)  [unwired: 1 in, 1 out]
                n158 = property on="Raw data values" class="MCListbox (엄격한)"(error in=w332) -> (error out=w334:errorcluster, "TopLeft"=w338:T9)  [unwired: 1 in, 1 out]
                n159 = Unbundle By Name(w338) -> ("Row"=w337:u32)
                n160 = Add(x=w337, y=w336) -> (x+y=w335:u64)
                n161 = property on="Raw data values" class="MCListbox (엄격한)"(error in=w334, "Value"=w335) -> (error out=w333:errorcluster)  [unwired: 1 in, 1 out]
              }
            }
          }
          event Key Down? {
            n162 = event-data() -> ("VKey"=w351:T11)  [unwired: 1 out]
            n163 = case shown="\"F1\"" w351 {
              tunnel: [FALSE ("Discard?") TRUE ("Discard?")] -> w350
              frame Default {
              }
              frame "F1" {
                n164 = call <vilib>:"TDMSFileViewer_LaunchHelp.vi"("CHM or HLP filename (lvdialog.chm)"="lvdialog.chm", "HTML filename"="tdms_file_viewer_db.html") -> ()  [unwired: 1 in, 5 out]
              }
            }
            n165 = event-data("Discard?"=w350) -> ()  [unwired: 1 in, 1 out]
          }
        }
      }
    }
    frame Error {
      n166 = call <vilib>:"Simple Error Handler.vi"("error in (no error)"=w358) -> ("error out"=w357:errorcluster)  [unwired: 1 in, 7 out]
    }
  }
  n167 = TDMS Close(8:w57, 11:w58) -> (0:w21:errorcluster)  [unwired: 1 out]
  n168 = case shown="참" w22 {
    tunnel: w21 -> [w360 w362]
    tunnel: [w360 w361] -> w8
    frame False {
    }
    frame True {
      n169 = invoke class="VI" method="FP.Close"(error in=w362) -> (error out=w361:errorcluster)  [unwired: 2 in, 2 out]
    }
  }
  n170 = Merge Errors(w6, w8) -> (→"error out":errorcluster)
